vi "Start.vi"(8 "error in (no error)":errorcluster, 11 "Analog Input in":refnum<class "Analog Input.lvclass">) -> (0 "error out":errorcluster, 3 "Analog Input out":refnum<class "Analog Input.lvclass">)   [LabVIEW 2009, in "MicroDAQ.lvlib" / "Analog Input.lvclass"]
doc: "Start acquisition. This VI must be used befor Read operation."
uses:
  <instrlib>/MicroDAQ/Channel/Analog Input/Analog Input.lvclass
  <instrlib>/MicroDAQ/Channel/Analog Input/Analog Input.lvclass/Analog Input.ctl
  <instrlib>/MicroDAQ/Channel/Channel.lvclass
  <instrlib>/MicroDAQ/Mlink library wraper/mlink.lvlib
  <instrlib>/MicroDAQ/MicroDAQ.lvlib
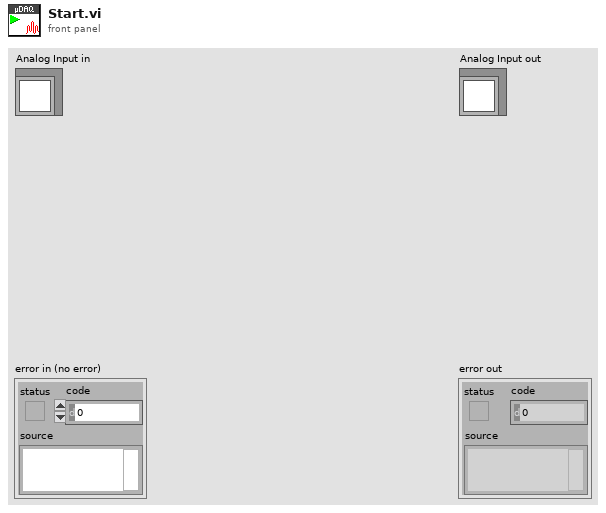
[diagram p1: front panel]
types:
  T1 = typedef "MicroDAQ.lvlib/Analo Range Enum.ctl" = enum16{"±10V", "0-10V", "±5V", "0-5V", "±5.12V", "±2.56V", "±2.5V", "±2V", "±1.24V", "±0.64V"}
  T2 = typedef "MicroDAQ.lvlib/Analog input type enum.ctl" = enum8{"Single-ended", "Differential"}
  T3 = typedef "MicroDAQ.lvlib/Analog input Channel enum.ctl" = u16
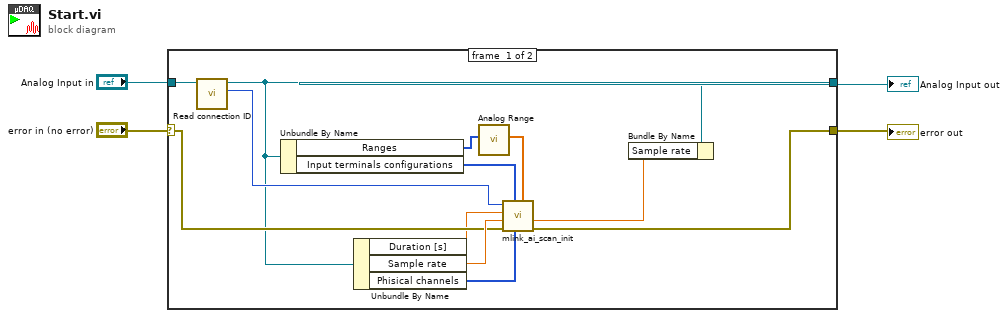
[diagram p0: block diagram]
diagram:
  n1 = case shown="No Error" "error in (no error)" {
    selector: "error in (no error)" -> [w10 w18]
    tunnel: "Analog Input in" -> [w17 w19]
    tunnel: [w7 w18] -> w2
    tunnel: [w8 w19] -> w1
    frame #0 {
      n2 = call <instrlib>:"Read connection ID.vi"("Task in"=w17) -> ("connection ID"=w9:i32, "Task out"=w5:refnum<class "Analog Input.lvclass">)  [unwired: 9 in]
      n3 = Unbundle By Name(w5) -> ("Ranges"=w12:T1[], "Input terminals configurations"=w11:T2[])
      n4 = Unbundle By Name(w5) -> ("Duration [s]"=w6:sgl, "Sample rate"=w14:sgl, "Phisical channels"=w15:T3[])
      n5 = call <instrlib>:"Analog Range.vi"("ranges in"=w12) -> ("range Array out"=w13:dbl[])  [unwired: 10 in]
      n6 = call <instrlib>:"mlink_ai_scan_init.vi"("range"=w13, "channels"=w15, "mode"=w11, "error in (no error)"=w10, "rate"=w14, "duration"=w6, "connection ID"=w9) -> ("error out"=w7:errorcluster, "actual rate"=w16:sgl)  [unwired: 2 in, 1 out]
      n7 = Bundle By Name(cluster=w5, "Sample rate"=w16) -> (w8:refnum<class "Analog Input.lvclass">)
    }
    frame #1 {
    }
  }
  "error out" <- w2
  "Analog Input out" <- w1
